vi "Uninit.vi"(11 "MuxActor in":refnum<class "MuxActor.lvclass">) -> (3 "MuxActor out":refnum<class "MuxActor.lvclass">)   [LabVIEW 2022 SP3, in "VideoMux.lvlib" / "MuxActor.lvclass"]
doc: "This method is the inverse of the Pre Launch Init.vi. This method is called unconditionally at the end of an actor's lifetime, even if there was an error in Pre Launch Init.vi. Note that the self Enqueuer for the actor is already invalid by the time this VI executes: within this method, the actor may send messages to its caller but not to itself. This method executes before Last Ack is sent.\n\nThis method neither receives nor produces an error cluster. It is designed to provide an unconditional release of acquired resources. Any error raised during release is considered to be irrelevant to the actor's lifetime. If the actor truly needs to report some error status, it may send a message to caller or include information within itself that callers can examine when handling Last Ack."
uses:
  MuxActor.lvclass
  MuxActor.lvclass/MuxActor.ctl
  Mux/Mux.lvclass
  <vilib>/ActorFramework/Actor/Actor.lvclass
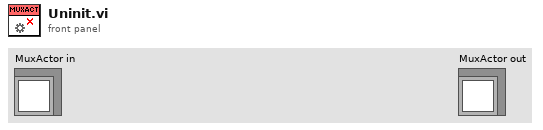
[diagram p1: front panel]
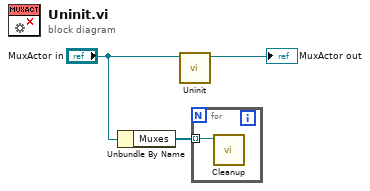
[diagram p0: block diagram]
diagram:
  n1 = Unbundle By Name("MuxActor in") -> ("Muxes"=w2:refnum<class "Mux.lvclass">[])
  n2 = call-parent "Uninit.vi"("Actor in"="MuxActor in") -> ("Actor out"=→"MuxActor out":refnum<class "MuxActor.lvclass">)  [unwired: 10 in]
  n3 = for {
    tunnel: w2 -> [w4] mode=indexing
    n4 = call-dynamic "Cleanup.vi"("Mux in"=w4) -> ()  [unwired: 10 in, 1 out]
  }
